vi "Process_BeamProfileGateSweep.vi"(0 "Refnum in":refnum<k34>, 1 "Acquire":bool, 2 "Capture number":i32, 5 "Gate Start":dbl, 7 "Gate Width":dbl, 9 "Image":dbl[][][](array[numeric]), 11 "error in (no error)":errorcluster, 12 "seconds since 1Jan1904":timestamp) -> (4 "Refnum out":refnum<k34>, 6 "Gate Delay Array":dbl[](array[numeric]), 8 "Avg Power each frame":dbl[](array[numeric]), 10 "Gate Delay of peak intensity":dbl, 15 "error out":errorcluster)   [LabVIEW 2017]
uses:
  <vilib>/Analysis/baseanly.llb/Mean (DBL).vi
  <vilib>/Analysis/NI_AALBase.lvlib
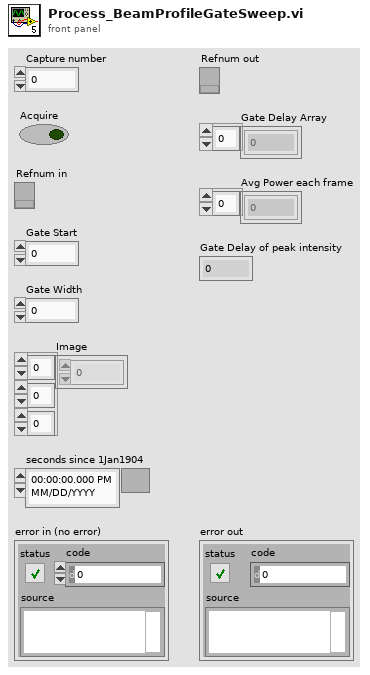
[diagram p1: front panel]
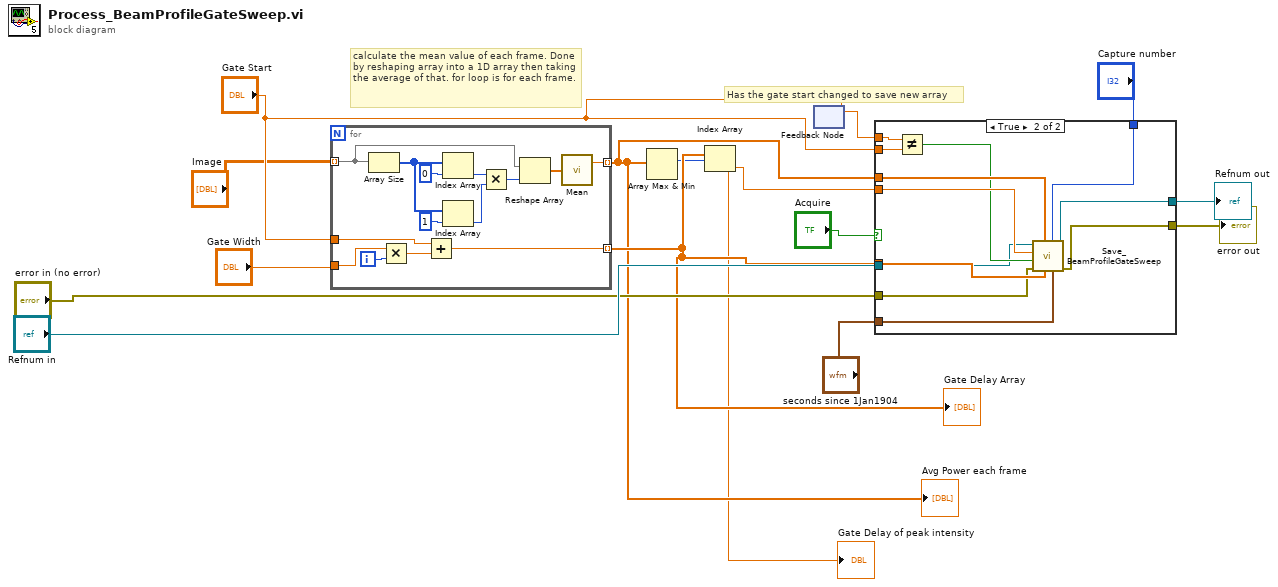
[diagram p0: block diagram]
diagram:
  # "Has the gate start changed to save new array"
  # "calculate the mean value of each frame. Done by reshaping array into a 1D array then taking the average of that. for loop is for each frame."
  n1 = for {
    tunnel: "Image" -> [w22] mode=indexing
    tunnel: [w29] -> w5 mode=indexing
    tunnel: "Gate Start" -> [w25]
    tunnel: "Gate Width" -> [w27]
    tunnel: [w24] -> w6 mode=indexing
    i -> [w28]
    n2 = Array Size(array=w22) -> (size(s)=w21:i32[])
    n3 = Multiply(x=w27, y=w28) -> (x*y=w26:dbl)
    n4 = Add(x=w25, y=w26) -> (x+y=w24:dbl)
    n5 = Index Array(array=w21, index=0) -> (element=w18:i32)
    n6 = Index Array(array=w21, index=1) -> (element=w17:i32)
    n7 = Multiply(x=w18, y=w17) -> (x*y=w16:i32)
    n8 = Reshape Array(w22, w16) -> (w23:dbl[])
    n9 = call-poly <vilib>:"Mean.vi"("X"=w23) -> ("mean"=w29:dbl)  [unwired: 1 out]
  }
  "Gate Delay Array" <- w6
  "Avg Power each frame" <- w5
  n10 = Array Max & Min(array=w5) -> (max index (indices)=w2:i32)  [unwired: 3 out]
  n11 = Index Array(array=w6, index=w2) -> (element=w3:dbl)
  "Gate Delay of peak intensity" <- w3
  n12 = feedback #1() -> (w9:dbl)  [unwired: 1 in]
  n13 = feedback-in #1("Gate Start") -> ()
  n14 = case shown="True" "Acquire" {
    tunnel: "seconds since 1Jan1904" -> [_ w38]
    tunnel: "Capture number" -> [_ w43]
    tunnel: w3 -> [_ w42]
    tunnel: w5 -> [_ w41]
    tunnel: w6 -> [_ w40]
    tunnel: w9 -> [_ w37]
    tunnel: "Gate Start" -> [_ w36]
    tunnel: [w30 w35] -> w12
    tunnel: [w31 w34] -> w13
    tunnel: "error in (no error)" -> [w30 w33]
    tunnel: "Refnum in" -> [w31 w32]
    frame False {
    }
    frame True {
      n15 = Not Equal?(x=w37, y=w36) -> (x != y?=w39:bool)
      n16 = call "Save_BeamProfileGateSweep.vi"("TimeStamp"=w38, "Capture Number"=w43, "Gate Delay Array"=w40, "Average power"=w41, "Error In"=w33, "Save new Gate delay array"=w39, "Gate Delay of peak intensity"=w42, "File In"=w32) -> ("error out"=w35:errorcluster, "File Out"=w34:refnum<k34>)  [unwired: 2 in]
    }
  }
  "Refnum out" <- w13
  "error out" <- w12
